vi "2.1.vi"() -> ()   [LabVIEW 2020]
panel:
  out "Elementos":dbl[](array[numeric])
  in  "Número de\nelementos":i32
  # "Serie Fibonacci"
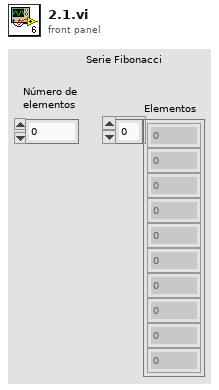
[diagram p1: front panel]
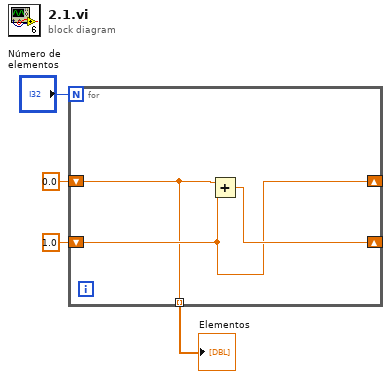
[diagram p0: block diagram]
diagram:
  n1 = for {
    N: "Número de\nelementos" -> [_]
    shift-right: [w6] -> _
    shift-left: 0.0 -> [w5]
    shift-right: [w7] -> _
    shift-left: 1.0 -> [w6]
    tunnel: [w5] -> w1 mode=indexing
    n2 = Add(x=w5, y=w6) -> (x+y=w7:dbl)
  }
  "Elementos" <- w1
